vi "Build and Execute RSSI Command.vi"(4 "Attenuation dB":dbl, 5 "2.45 GHz Wake-Up Power":i8(ring)=6 items=["-29"=-29, "-4"=-4, "-2"=-2, "0"=0, "2"=2, "4"=4, "6"=6, "8"=8, "10"=10, "12"=12, "14"=14, "16"=16, "18"=18, "20"=20, "22"=22, "24"=24, "26"=26, "27"=27], 6 "400 MHz MICS Power Setting":u8=22 format="%.0x", 7 "Channel (for RSSI Measurement)":u8=255, 8 "error in":errorcluster, 9 "Duration (for RSSI Measurement)":u16=100, 10 "Delay (for RSSI Measurement)":u16=100, 11 "VISA resource in":refnum<visa-resource-name>) -> (0 "error out":errorcluster, 3 "dup VISA resource":refnum<visa-resource-name>)   [LabVIEW 2010]
uses:
  Typedef Command List.ctl
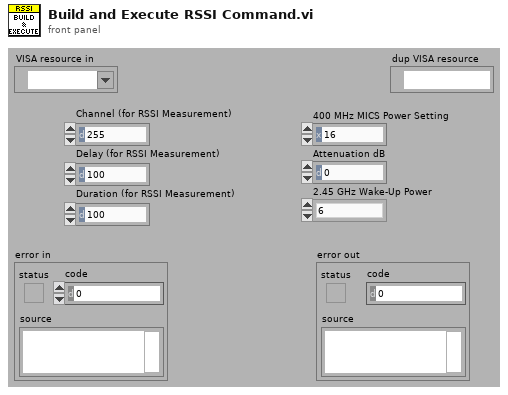
[diagram p1: front panel]
types:
  T1 = typedef "Typedef Command List.ctl" = enum16{"Get xPG Status", "xPG Stimulation", "Select Program", "Increment Program Amplitude", "Decrement Program Amplitude", "Get PoP Constants", "Get PPC Constants", "Get Program Names", "Set Pulse Amplitude", "Increment Pulse Amplitude", "Decrement Pulse Amplitude", "Get Pulse Widths", "Set Pulse Widths", "Increment Pulse Width", "Decrement Pulse Width", "Get Program Frequency", "Set Program Frequency", "Increment Program Frequency", "Decrement Program Frequency", "Inject Event", "Charging Control", "Get xPG Identity", "Set xPG Identity", "Restore Program Defaults", "Get Program Definition", "Set Program Definition", "Get Program Constants", "Set Program Constants", "Get Configurable Device Parameters", "Set Configurable Device Parameters", "Get Pulse Constants", "Set Pulse Constants", "Get Lead Limits", "Set Lead Limits", "Get Channel Calibrations", "Set Channel Calibrations", "<reserved 2>", "<reserved 3>", "<reserved 4>", "<reserved 5>", "<reserved 6>", "<reserved 7>", "Get Stim Asic HV Calibrations", "Set Stim Asic HV Calibrations", "<reserved 8>", "<reserved 9>", "Get CP Data", "Set CP Data", "Clear Log", "Read Log", "Append Log", "Get Patient Program Runtime", "Set Patient Program Runtime", "Impedance Measurement", "Enter Storage Mode", "Echo Short", "Echo Long", "Get General Calibration", "Set General Calibration", "Get Trim List", "Set Trim List", "Get Counter", "Set Counter", "Get Test Stimulation", "Set Test Stimulation", "Get Titration Stimulation", "Set Titration Stimulation", "Get Ramp Time", "Set Ramp Time", "Get VBAT", "Set Software Description Block", "Get Software Description Block", "Write Memory", "Read Memory", "Reset xPG", "Erase Flash Block", "Write Vectors", "Read Vectors", "Diagnostic Data", "Set Background Impedance", "Get Background Impedence ", "Set Test Waveform", "Calibrate Channel", "Get Log Range", "Reserved 0x55", "Reserved 0x56", "MICS Options", "Pair PPC", "Pair POP", "Stop Bootloader", "Tune MICS", "MICS Diagnostics", "Undefined"}
  T2 = cluster{"Command":T1, "Function":enum16{"Open Session", "Close Session", "Downlink Only", "Uplink Only", "Transceive (DN -> UP)"}, "MICS_ID":u32, "EXID":u32, "Use Local":bool, "Transceive Delay mS":dbl, "CP_DATA IN":u8[], "Parameters":string}
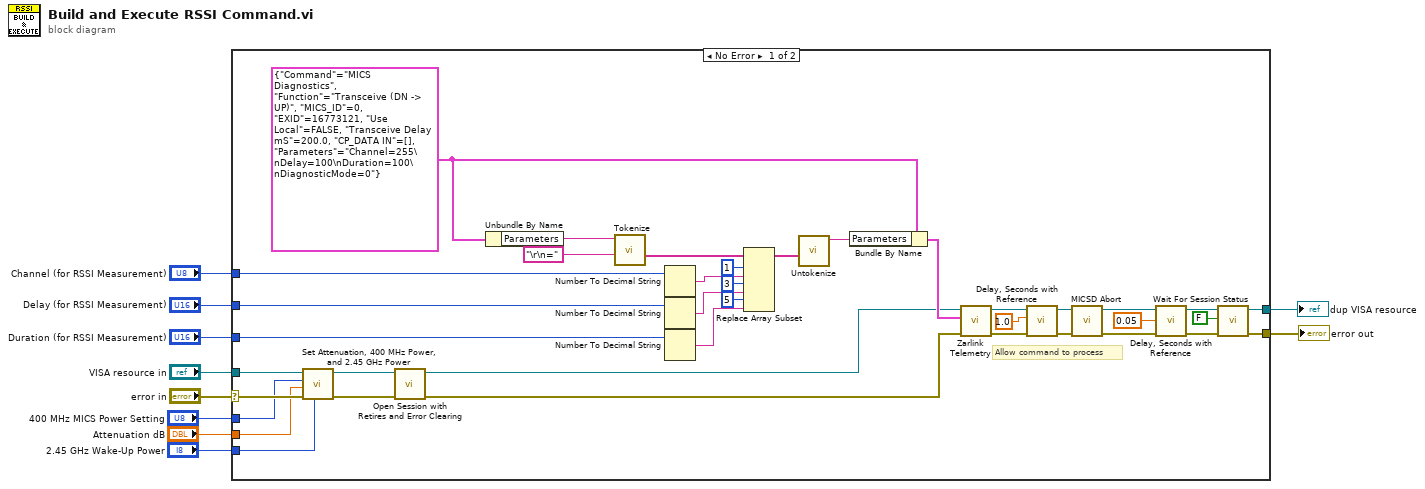
[diagram p0: block diagram]
diagram:
  n1 = case shown="No Error" "error in" {
    selector: "error in" -> [w29 w49]
    tunnel: "VISA resource in" -> [w27 w48]
    tunnel: [w19 w49] -> w9
    tunnel: "Channel (for RSSI Measurement)" -> [w35 _]
    tunnel: "Delay (for RSSI Measurement)" -> [w34 _]
    tunnel: "Duration (for RSSI Measurement)" -> [w33 _]
    tunnel: [w18 w48] -> w4
    tunnel: "400 MHz MICS Power Setting" -> [w26 _]
    tunnel: "Attenuation dB" -> [w25 _]
    tunnel: "2.45 GHz Wake-Up Power" -> [w17 _]
    frame No Error {
      w39 = T2 {"Command"=enum."MICS Diagnostics", "Function"=enum."Transceive (DN -> UP)", "MICS_ID"=0, "EXID"=16773121, "Use Local"=FALSE, "Transceive Delay mS"=200.0, "CP_DATA IN"=[], "Parameters"="Channel=255\nDelay=100\nDuration=100\nDiagnosticMode=0"} ("Input")
      # "Allow command to process"
      n2 = call "Set Attenuation, 400 MHz Power, and 2.45 GHz Power.vi"("2.45 GHz Wake-Up Power (6)"=w17, "error in"=w29, "Attenuation dB (0)"=w25, "400 MHz MICS Power Setting (0x16)"=w26, "VISA Resource Name"=w27) -> ("error out"=w30:errorcluster, "dup VISA Resource Name"=w31:refnum<visa-resource-name>)  [unwired: 5 in]
      n3 = call "Open Session with Retires and Error Clearing.vi"("error in"=w30, "VISA Resource Name"=w31) -> ("error out"=w28:errorcluster, "dup VISA Resource Name"=w16:refnum<visa-resource-name>)  [unwired: 6 in, 2 out]
      n4 = Unbundle By Name(w39) -> ("Parameters"=w47:string)
      n5 = call "Tokenize.vi"("delimiters (\\s,\\t,\\r,\\n,=)"="\r\n=" ("delimiters (\\s,\\t,\\r,\\n,=)"), "input string"=w47) -> ("tokens"=w46:string[])  [unwired: 3 in, 2 out]
      n6 = Number To Decimal String(number=w35) -> (decimal integer string=w38:string)  [unwired: 1 in]
      n7 = Number To Decimal String(number=w34) -> (decimal integer string=w37:string)  [unwired: 1 in]
      n8 = Number To Decimal String(number=w33) -> (decimal integer string=w36:string)  [unwired: 1 in]
      n9 = Replace Array Subset(array=w46, new element #1=w38, index #1=1 ("index"), new element #2=w37, index #2=3 ("index"), new element #3=w36, index #3=5 ("index")) -> (w41:string[])
      n10 = call "Untokenize.vi"("tokens"=w41) -> ("string out"=w40:string)  [unwired: 10 in]
      n11 = Bundle By Name(cluster=w39, "Parameters"=w40) -> (w32:T2)
      n12 = call "Zarlink Telemetry.vi"("error in (no error)"=w28, "Input"=w32, "MICS Dongle Address"=w16) -> ("error out"=w21:errorcluster)  [unwired: 6 in, 2 out]
      n13 = call "Delay, Seconds with Reference.vi"("error in"=w21, "delay"=dbl[unit] 1.0, "VISA resource"=w16) -> ("error out"=w24:errorcluster, "VISA resource dup"=w23:refnum<visa-resource-name>)  [unwired: 3 in, 1 out]
      n14 = call "MICSD Abort.vi"("error in (no error)"=w24, "VISA Resource Name"=w23) -> ("error out"=w13:errorcluster, "dup VISA Resource Name"=w15:refnum<visa-resource-name>)  [unwired: 8 in]
      n15 = call "Delay, Seconds with Reference.vi"("error in"=w13, "delay"=dbl[unit] 0.05, "VISA resource"=w15) -> ("error out"=w12:errorcluster, "VISA resource dup"=w14:refnum<visa-resource-name>)  [unwired: 3 in, 1 out]
      n16 = call "Wait For Session Status.vi"("error in (no error)"=w12, "IN_SESSION State (T)"=FALSE, "VISA Resource Name"=w14) -> ("error out"=w19:errorcluster, "dup VISA Resource Name"=w18:refnum<visa-resource-name>)  [unwired: 5 in, 2 out]
    }
    frame Error {
    }
  }
  "error out" <- w9
  "dup VISA resource" <- w4
